vi "extract timing from header start.vi"(7 "Header String":string="Npts = 8192\nRate = 2048 Hz") -> (2 "Rate (Hz)":dbl, 8 "Interval (s)":dbl)   [LabVIEW 2019]
doc: "This subvi extracts the rate from a file header; it also calculates the time interval by inverting the rate."
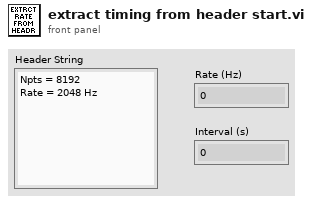
[diagram p1: front panel]
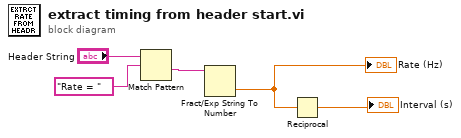
[diagram p0: block diagram]
diagram:
  n1 = Match Pattern(string="Header String", regular expression="Rate = ") -> (after substring=w2:string)  [unwired: 1 in, 3 out]
  n2 = Fract/Exp String To Number(string=w2) -> (number=w1:dbl)  [unwired: 3 in, 1 out]
  "Rate (Hz)" <- w1
  n3 = Reciprocal(x=w1) -> (1/x=→"Interval (s)":dbl)
